vi "KE622x -- 2182 -A Set Range.vi"(0 "622x Resource In":refnum<visa-resource-name>, 1 "Check For SCPI Errors? (T)":bool=TRUE, 7 "2182/2182A Range":T1, 11 "error in (no error)":errorcluster) -> (4 "622x Resource Out (dupl)":refnum<visa-resource-name>, 15 "error out":errorcluster)   [LabVIEW 2019, in "Keithley 622x.lvlib"]
uses:
  Keithley 622x.lvlib
  Typedefs/KE2182 -- Voltage Ranges.ctl
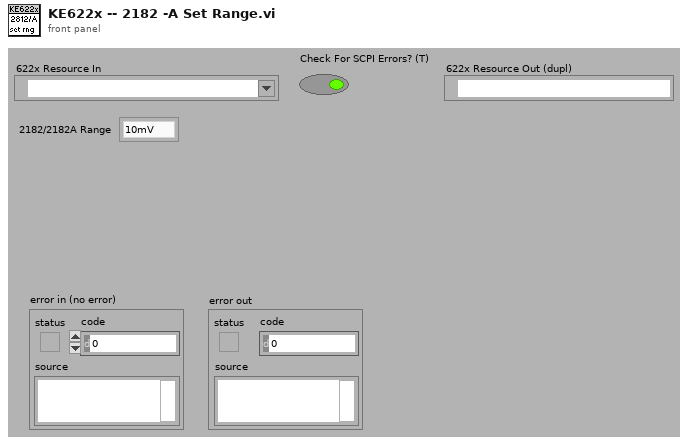
[diagram p1: front panel]
types:
  T1 = typedef "Keithley 622x.lvlib/KE2182 -- Voltage Ranges.ctl" = enum16{"10mV", "100mV", "1V", "10V", "100V"}
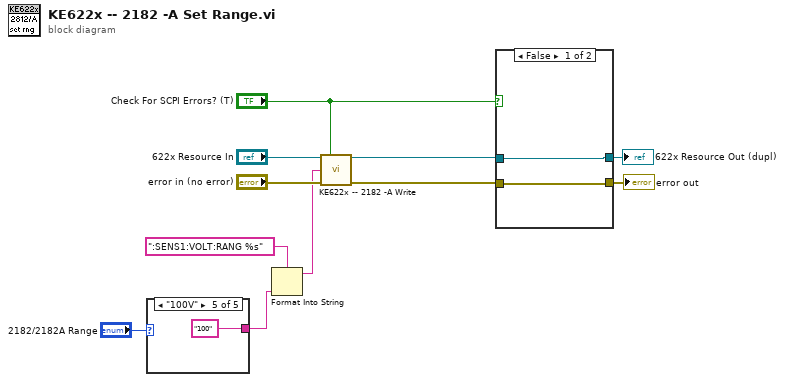
[diagram p0: block diagram]
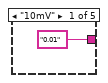
[diagram p2: hidden frame]
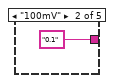
[diagram p3: hidden frame]
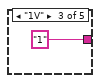
[diagram p4: hidden frame]
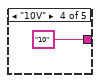
[diagram p5: hidden frame]
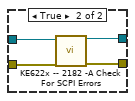
[diagram p6: hidden frame]
diagram:
  n1 = case shown="\"100V\"" "2182/2182A Range" {
    tunnel: ["0.01" "0.1" "1" "10" "100"] -> w3
    frame "10mV" {
    }
    frame "100mV" {
    }
    frame "1V" {
    }
    frame "10V" {
    }
    frame "100V" {
    }
  }
  n2 = Format Into String(format string=":SENS1:VOLT:RANG %s", w3) -> (resulting string=w2:string)  [unwired: 2 in, 1 out]
  n3 = call "KE622x -- 2182 -A Write.vi"("Resource In"="622x Resource In", "Check For SCPI Errors? (T)"="Check For SCPI Errors? (T)", "2182-A Write String"=w2, "error in (no error)"="error in (no error)") -> ("Resource Out (dupl)"=w9:refnum<visa-resource-name>, "error out"=w1:errorcluster)  [unwired: 10 in]
  n4 = case shown="False" "Check For SCPI Errors? (T)" {
    tunnel: w9 -> [w18 w22]
    tunnel: w1 -> [w17 w21]
    tunnel: [w18 w20] -> w7
    tunnel: [w17 w19] -> w6
    frame False {
    }
    frame True {
      n5 = call "KE622x -- 2182 -A Check For SCPI Errors.vi"("VISA Resource In"=w22, "error in (no error)"=w21) -> ("VISA Resource Out (dupl)"=w20:refnum<visa-resource-name>, "error out"=w19:errorcluster)  [unwired: 10 in, 2 out]
    }
  }
  "622x Resource Out (dupl)" <- w7
  "error out" <- w6
